vi "test_nmea_replay.vi"() -> ()   [LabVIEW 2019]
panel:
  in  "dt":u32
  out "n":i32
  out "XY 그래프":cluster{"X":dbl, "Y":dbl}[](graph)
  in  "path":path=path "C:/Users/WEGO/Documents/GitHub/Ycar/LabVIEW/GPS/logfile/nmea-anyang-beomgye.txt"
  out "latlong":cluster{"Lat":dbl, "Long":dbl} {"Lat" format="%.8f"; "Long" format="%.8f"}
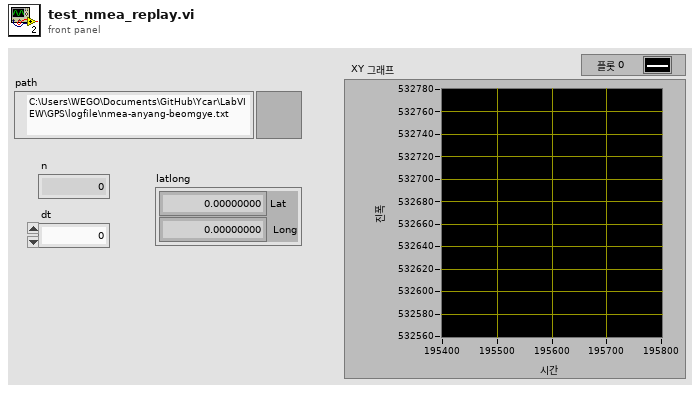
[diagram p1: front panel]
types:
  T1 = enum16{"GxDTM", "GxGBS", "GxGGA", "GxGLL", "GxGNS", "GxGRS", "GxGSA", "GxGST", "GxGSV", "GxRLM", "GxRMC", "GxTHS", "GxTXT", "GxVLW", "GxVTG", "GxZDA"}
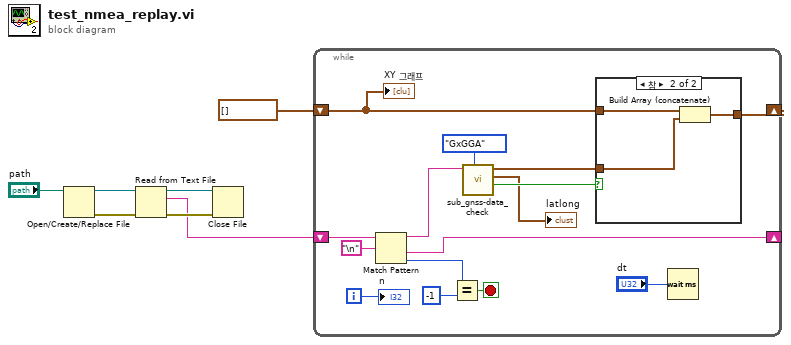
[diagram p0: block diagram]
diagram:
  n1 = Open/Create/Replace File(file path (use dialog)="path") -> (refnum out=w4:refnum<file>, error out=w7:errorcluster)  [unwired: 5 in, 1 out]
  n2 = Read from Text File(file (use dialog)=w4, error in=w7) -> (refnum out=w5:refnum<file>, text=w1:string, error out=w6:errorcluster)  [unwired: 2 in, 1 out]
  n3 = Close File(refnum=w5, error in=w6) -> ()  [unwired: 2 out]
  n4 = while {
    shift-right: [w19] -> _
    shift-left: cluster{"Lat":dbl, "Long":dbl}[] [] -> [w15]
    shift-right: [w18] -> _
    shift-left: w1 -> [w14]
    i -> [w17]
    stop <- w20 stop-if-true
    n5 = Match Pattern(string=w14, regular expression="\n") -> (before substring=w11:string, after substring=w18:string, offset past match=w13:i32)  [unwired: 1 in, 1 out]
    n6 = Equal?(x=w13, y=-1) -> (x = y?=w20:bool)
    n7 = call "sub_gnss-data_check.vi"("sel"=T1."GxGGA", "gnss str"=w11) -> ("val"=w10:bool, "LatLong"=→"latlong":cluster{dbl, dbl}, "TM"=w8:cluster{dbl, dbl})  [unwired: 6 in, 1 out]
    n8 = case shown="참" w10 {
      tunnel: [w23 w26] -> w19
      tunnel: w15 -> [w23 w25]
      tunnel: w8 -> [_ w24]
      frame False {
      }
      frame True {
        n9 = Build Array (concatenate)(w25, w24) -> (w26:cluster{"Lat":dbl, "Long":dbl}[])
      }
    }
    n10 = Wait (ms)(milliseconds to wait="dt") -> ()  [unwired: 1 out]
    "n" <- w17
    "XY 그래프" <- w15
  }
